vi "仁莫密封检测系统.vi"() -> ()   [LabVIEW 2020]
uses:
  <vilib>/event_ctls.llb/eventvkey.ctl
  <vilib>/NI/Modbus Library/API/Master/Modbus Master.lvclass
  <vilib>/Utility/file.llb/Read Delimited Spreadsheet (string).vi
  <vilib>/NI/Modbus Library/Transmission Data Unit/RTU/RTU Data Unit.lvclass
  <vilib>/NI/Modbus Library/Master Function Definition/Master Function Definition.lvclass
  <vilib>/NI/Modbus Library/Network Protocol/Network Master/Serial/Serial Master.lvclass
panel:
  in  "sn":string
  in  "扫码启动":bool
  out "MES状态":bool
  out "通讯状态":bool
  out "泄漏流量":string
  out "参数组别":string
  out "测试时间":string
  out "实时压力":string
  out "泄漏压力":string
  out "门限压力":string
  out "目标压力":string
  out "测试 NG":string
  out "测试 OK":string
  out "测试结果":string
  out "测试总量":string
  out "实时压力(图)":dbl(graph)
  out "消息框+":string
  in  "清除计数":bool
  in  "设备启动":bool
  out "运行状态":string
  in  "设备停止":bool
  in  "阻断通讯":bool=TRUE
  out "运行状态":string
  out "失败原因":string
  in  "Exit":bool
  # "仁 莫 密 封 检 测 系 统"
  # "sccm"
  # "S"
  # "Pa"
  # "Pa"
  # "Pa"
  # "Pa"
  # "pcs"
  # "pcs"
  # "pcs"
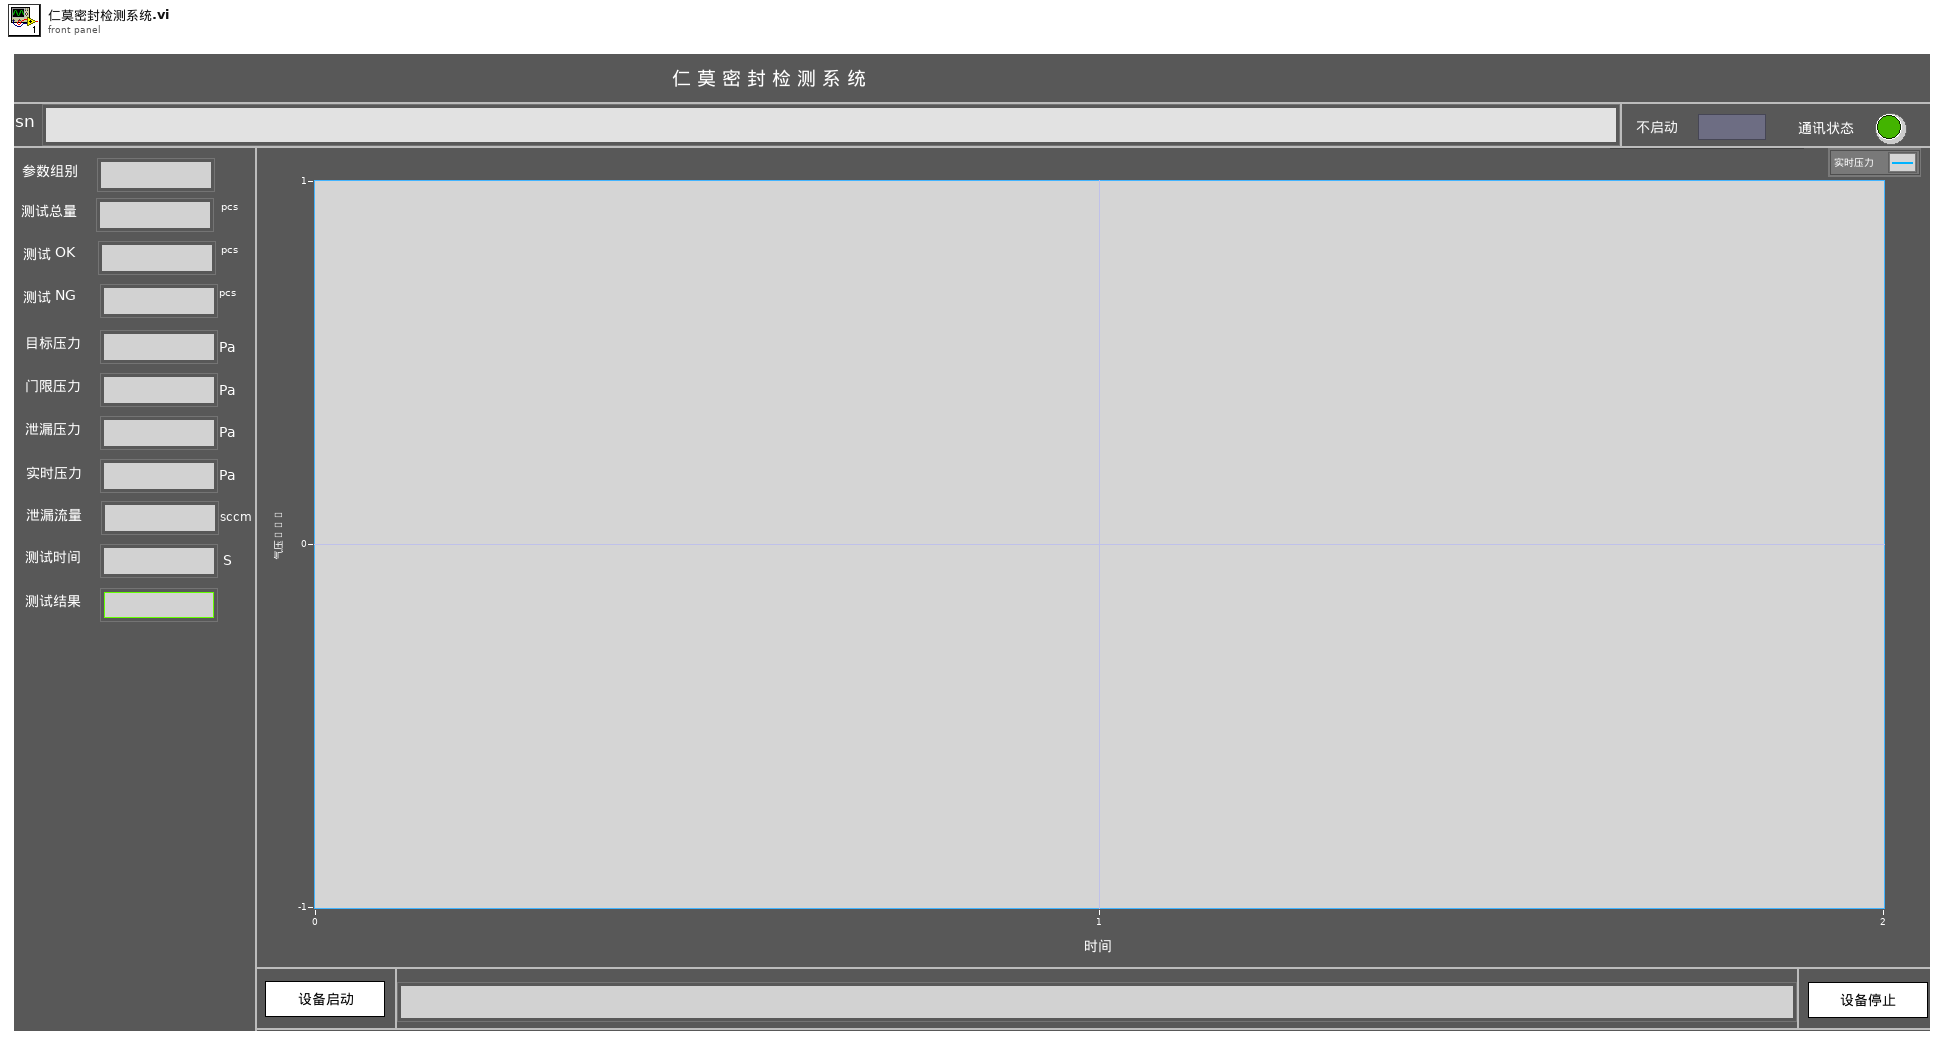
[diagram p1: front panel]
types:
  T1 = typedef "eventvkey.ctl" = enum16{"ASCII", "Enter", "Return", "Shift", "Ctrl", "Alt", "Cmd", "Opt", "Caps", "NumLock", "Clear", "Break", "Up", "Down", "Left", "Right", "Insert", "Delete", "Home", "End", "PageUp", "PageDown", "Escape", "Help", "Pause", "ScrollLock", "F1", "F2", "F3", "F4", "F5", "F6", "F7", "F8", "F9", "F10", "F11", "F12", "F13", "F14", "F15", "F16", "F17", "F18", "F19", "F20", "F21", "F22", "F23", "F24", "Play", "VolumeUp", "VolumeDown", "Mute", "Two Byte Char"}
  T2 = cluster{"地址":u16, "数量":u16, "寄存器值":u16[], "产品总数":string}[]
  T3 = enum32{"Invalid", "Standard", "Closed", "Hidden", "Minimized", "Maximized"}
  T4 = enum32{"invalid app kind", "Development System", "Run Time System", "Student Edition", "Embedded LabVIEW", "Evaluation", "Custom"}
  T5 = cluster{"地址":u16, "数量":u16, "寄存器值":u16[], "名称":string}[]
  T6 = cluster{"读取信息簇":cluster{"地址":u16, "数量":u16, "寄存器值":u16[], "名称":string}, "值解析":string}[]
  T7 = cluster{"温度instance":refnum<class "Modbus Master.lvclass">, "Core":cluster{"Current VI Reference":refnum<vi>, "Close Panel on Exit?":bool}, "serial master instance":refnum<class "Modbus Master.lvclass">, "进站OK":bool, "连接成功":bool, "正在运行":bool, "用户登录":bool, "A读保持寄存器信息组":cluster{"地址":u16, "数量":u16, "寄存器值":u16[], "名称":string}[], "A写入线圈信息组":cluster{"地址":u16, "布尔":bool, "名称":string}[], "A读多组线圈信息组":cluster{"地址":u16, "数量":u16, "名称":string, "线圈组":bool[]}[]}
  T8 = cluster{"连接成功":bool, "MB_实体":refnum<class "Modbus Master.lvclass">}
  T9 = cluster{"地址":u16, "数量":u16, "名称":string, "线圈组":bool[]}[]
  T10 = cluster{"Current VI Reference":refnum<vi>, "Close Panel on Exit?":bool}
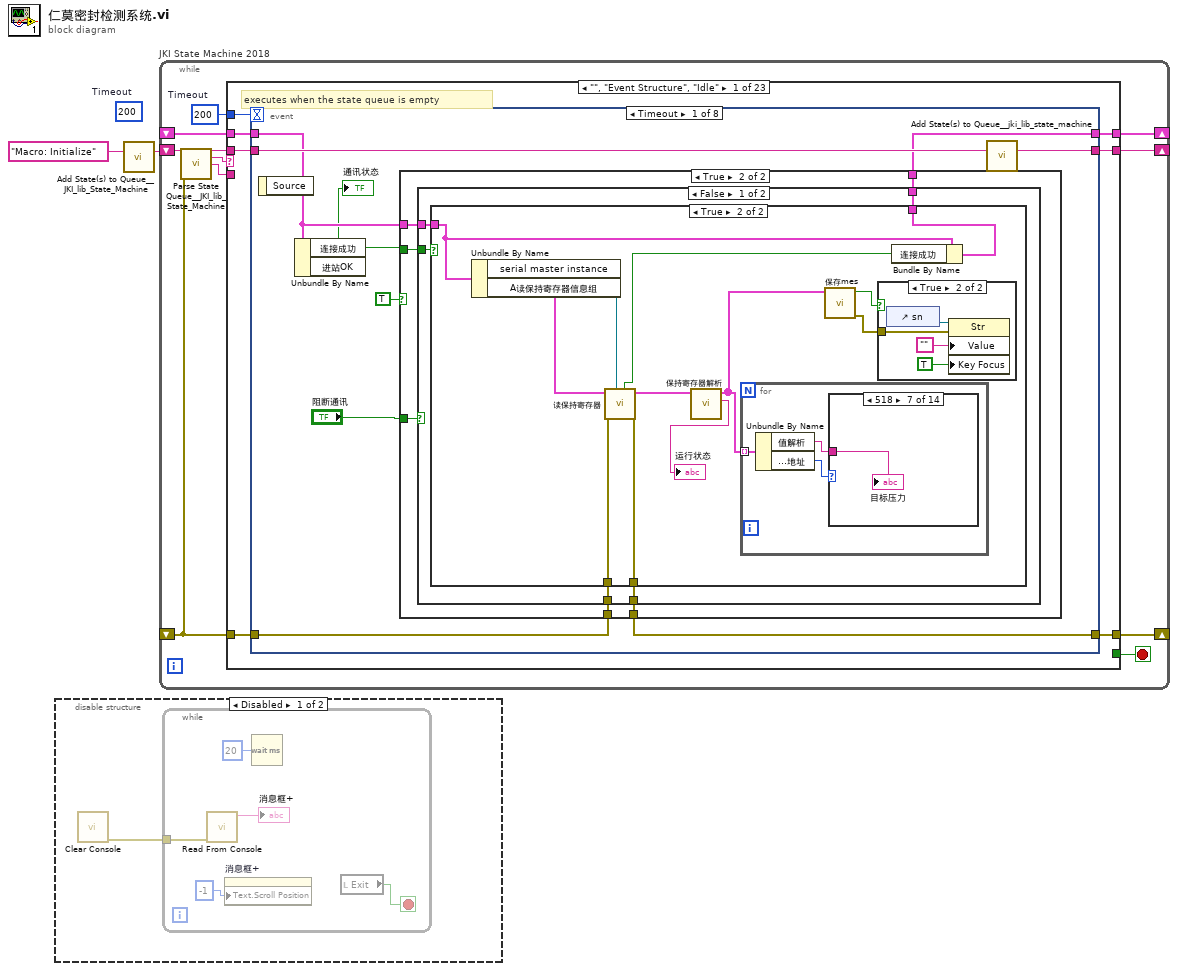
[diagram p0: block diagram]
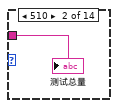
[diagram p7: hidden frame]
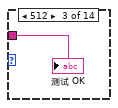
[diagram p8: hidden frame]
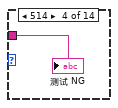
[diagram p9: hidden frame]
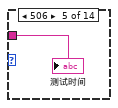
[diagram p10: hidden frame]
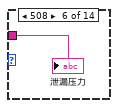
[diagram p11: hidden frame]
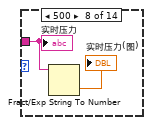
[diagram p12: hidden frame]
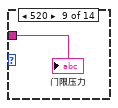
[diagram p13: hidden frame]
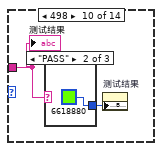
[diagram p14: hidden frame]
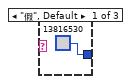
[diagram p15: hidden frame]
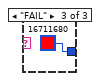
[diagram p16: hidden frame]
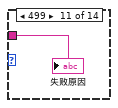
[diagram p17: hidden frame]
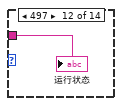
[diagram p18: hidden frame]
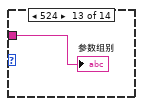
[diagram p19: hidden frame]
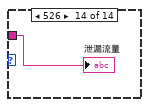
[diagram p20: hidden frame]
diagram:
  (unwired) 200  # Timeout
  n1 = disable-structure shown="Disabled" {
    frame Disabled {
      n2 = call "Clear Console.vi"() -> ("error out"=w3:errorcluster)  [unwired: 11 in]
      n3 = while {
        tunnel: w3 -> [w7]
        stop <- w4 stop-if-true
        n4 = call "Read From Console.vi"("error in (no error)"=w7) -> ("Output"=→"消息框+":string)  [unwired: 9 in, 1 out]
        n5 = property on="消息框+" class="Str"("Text.Scroll Position"=i8 -1 ("milliseconds to wait")) -> ()  [unwired: 2 in, 2 out]
        n6 = Wait (ms)(milliseconds to wait=u32 20 ("等待时间（毫秒）")) -> ()  [unwired: 1 out]
        n7 = local read "Exit"() -> (w4:bool)
      }
    }
    frame Enabled {
    }
  }
  n8 = call <vilib>:"Add State(s) to Queue__JKI_lib_State_Machine.vi"("State(s) in (\"\")"="Macro: Initialize") -> ("States Out"=w2:string)  [unwired: 14 in]
  n9 = while "JKI State Machine 2018" {
    shift-right: [w12] -> _
    shift-left: _ -> [w11]
    shift-right: [w15] -> _
    shift-left: _ -> [w9]
    shift-right: [w14] -> _
    shift-left: w2 -> [w16]
    stop <- w13 stop-if-true
    w10 = 200  # Timeout
    n10 = call <vilib>:"Parse State Queue__JKI_lib_State_Machine.vi"("State Queue"=w16, "Error In (no error)"=w9) -> ("Remaining States"=w18:string, "Current State"=w19:string, "Arguments"=w17:string)  [unwired: 11 in]
    n11 = case shown="\"\", \"Event Structure\", \"Idle\"" w19 {
      selector: w19 -> [_ _ w199 _ _ _ _ _ _ _ _ _ _ _ _ _ _ _ _ _ _ _ _]
      tunnel: w18 -> [w26 w198 w203 w222 w229 w234 w238 w263 w272 w276 w293 w299 w310 w379 w384 w394 w398 w410 w422 w469 w501 w513 w518]
      tunnel: w17 -> [_ _ _ _ _ _ _ _ _ _ _ w294 w304 _ _ _ _ _ _ _ _ _ _]
      tunnel: w11 -> [w24 w195 w201 w215 w226 w232 w235 _ w268 w273 w291 w297 w306 w376 w381 w391 w395 w404 w416 w463 w494 w510 w515]
      tunnel: [w23 w196 w205 w219 errorcluster {"status"=FALSE, "code"=0, "source"=""} ("error out") w231 w236 w260 w269 w274 w290 w295 w307 w377 w382 w392 w396 w399 w419 w466 w498 w511 w516] -> w15
      tunnel: w9 -> [w22 w196 w204 w219 w224 w231 w236 w260 w266 w274 w290 w296 w308 w377 w382 w392 w396 w407 w420 w467 w499 w511 w516]
      tunnel: [w25 w197 w202 w221 w228 w233 w237 w262 w271 w275 w292 w298 w309 w378 w383 w393 w397 w409 w421 w468 w500 w512 w517] -> w14
      tunnel: [_ _ _ _ _ w230 _ _ _ _ _ _ _ _ _ _ _ _ _ _ _ _ _] -> w13
      tunnel: [w21 w195 w201 w220 w226 w232 w235 w261 w268 w273 w291 w297 w306 w376 w381 w391 w395 w402 w414 w461 w495 w510 w514] -> w12
      tunnel: w10 -> [w20 _ _ _ _ _ _ _ _ _ _ _ _ _ _ _ _ _ _ _ _ _ _]
      frame "", "Event Structure", "Idle" {
        # "executes when the state queue is empty"
        n12 = event shown="[0] Timeout" {
          selector: _ -> [_ _ _ _ _ _ _ _]
          dyn-events: _ -> [_ _ _ _ _ _ _ _]
          timeout: w20 -> [_ _ _ _ _ _ _ _]
          tunnel: w26 -> [w35 w94 w99 w105 w159 w178 w188 w194]
          tunnel: [w34 w93 w98 w104 w158 w177 w187 w193] -> w25
          tunnel: w24 -> [w33 w91 w96 w101 w156 w173 w185 w191]
          tunnel: [w31 w92 w97 w103 w157 w170 w186 w192] -> w23
          tunnel: w22 -> [w32 w92 w97 w103 w157 w171 w186 w192]
          tunnel: [w30 w91 w96 w100 w156 w172 w185 w191] -> w21
          event Timeout {
            n13 = event-data() -> ()  [unwired: 1 in, 1 out]
            n14 = Unbundle By Name(w33) -> ("连接成功"=w27:bool)  [unwired: 1 out]
            "通讯状态" <- w27
            n15 = case shown="True" TRUE {
              tunnel: w33 -> [w37 w43]
              tunnel: w32 -> [w36 w42]
              tunnel: [w36 w41] -> w31
              tunnel: [w37 w40] -> w30
              tunnel: "阻断通讯" -> [_ w39]
              tunnel: w27 -> [_ w38]
              frame False {
              }
              frame True {
                n16 = case shown="False" w39 {
                  tunnel: w38 -> [w48 _]
                  tunnel: w43 -> [w47 w88]
                  tunnel: w42 -> [w46 w89]
                  tunnel: [w45 w89] -> w41
                  tunnel: [w44 w88] -> w40
                  frame False {
                    n17 = case shown="True" w48 {
                      tunnel: w47 -> [w49 w60]
                      tunnel: w46 -> [w50 w62]
                      tunnel: [w50 w61] -> w45
                      tunnel: [w49 w55] -> w44
                      frame False {
                      }
                      frame True {
                        n18 = Unbundle By Name(w60) -> ("serial master instance"=w59:refnum<class "Modbus Master.lvclass">, "A读保持寄存器信息组"=w58:T5)
                        n19 = call "读保持寄存器.vi"("MB_实体"=w59, "error in"=w62, "读保持寄存器信息组__输入"=w58) -> ("输出簇"=w61:errorcluster, "读保持寄存器信息组_输出"=w56:T5, "连接成功"=w57:bool)  [unwired: 6 in]
                        n20 = call "保持寄存器解析.vi"("A读保持寄存器信息组"=w56) -> ("运行状态"=→"运行状态":string, "参数值"=w54:T6)  [unwired: 9 in]
                        n21 = for {
                          tunnel: w54 -> [w68] mode=indexing
                          n22 = Unbundle By Name(w68) -> ("值解析"=w67:string, "读取信息簇.地址"=w69:u16)
                          n23 = case shown="518" w69 {
                            tunnel: w67 -> [_ w70 w71 w72 w73 w74 w75 w77 w78 w80 w84 w85 w86 w87]
                            frame Default {
                            }
                            frame 510 {
                              "测试总量" <- w70
                            }
                            frame 512 {
                              "测试 OK" <- w71
                            }
                            frame 514 {
                              "测试 NG" <- w72
                            }
                            frame 506 {
                              "测试时间" <- w73
                            }
                            frame 508 {
                              "泄漏压力" <- w74
                            }
                            frame 518 {
                              "目标压力" <- w75
                            }
                            frame 500 {
                              n24 = Fract/Exp String To Number(string=w77) -> (number=→"实时压力(图)":dbl)  [unwired: 3 in, 1 out]
                              "实时压力" <- w77
                            }
                            frame 520 {
                              "门限压力" <- w78
                            }
                            frame 498 {
                              n25 = case shown="\"PASS\"" w80 {
                                tunnel: [u32 13816530 ("颜色盒") u32 6618880 u32 16711680] -> w79
                                frame "假", Default {
                                }
                                frame "PASS" {
                                }
                                frame "FAIL" {
                                }
                              }
                              n26 = property on="测试结果" class="Str"("Text.BGColor"=w79) -> ()  [unwired: 2 in, 2 out]
                              "测试结果" <- w80
                            }
                            frame 499 {
                              "失败原因" <- w84
                            }
                            frame 497 {
                              "运行状态" <- w85
                            }
                            frame 524 {
                              "参数组别" <- w86
                            }
                            frame 526 {
                              "泄漏流量" <- w87
                            }
                          }
                        }
                        n27 = call "保存mes.vi"("参数值"=w54) -> ("error out"=w52:errorcluster, "出站成功"=w51:bool)  [unwired: 9 in]
                        n28 = case shown="True" w51 {
                          tunnel: w52 -> [_ w65]
                          frame False {
                          }
                          frame True {
                            n29 = control-ref of="sn"() -> (w66:refnum<vi>)
                            n30 = property on="属性节点" class="Str"(reference=w66, error in=w65, "Value"="", "Key Focus"=TRUE ("键选中")) -> ()  [unwired: 2 out]
                          }
                        }
                        n31 = Bundle By Name(cluster=w60, "连接成功"=w57) -> (w55:T7)
                      }
                    }
                  }
                  frame True {
                  }
                }
              }
            }
            n32 = call <vilib>:"Add State(s) to Queue__jki_lib_state_machine.vi"("State(s) in (\"\")"=w35) -> ("States Out"=w34:string)  [unwired: 14 in]
          }
          event "设备启动": Value Change {
            n33 = event-data() -> ()  [unwired: 1 in, 1 out]
            n34 = call <vilib>:"Add State(s) to Queue__jki_lib_state_machine.vi"("State(s) in Front (\"\")"="//Communication: 读运行标志\nCommunication: 设备启动\n//Communication: 读运行标志", "State(s) in (\"\")"=w94) -> ("States Out"=w93:string)  [unwired: 13 in]
          }
          event "设备停止": Value Change {
            n35 = event-data() -> ()  [unwired: 1 in, 1 out]
            n36 = call <vilib>:"Add State(s) to Queue__jki_lib_state_machine.vi"("State(s) in Front (\"\")"="//Communication: 读运行标志\nCommunication: 设备停止\n//Communication: 读运行标志", "State(s) in (\"\")"=w99) -> ("States Out"=w98:string)  [unwired: 13 in]
          }
          event Menu Selection (User) {
            n37 = event-data() -> ("ItemTag"=w102:string)  [unwired: 1 in]
            n38 = case shown="\"历史数据路径配置\"" w102 {
              tunnel: w101 -> [w106 w107 w118 w129 w130 w132 w143 w151]
              tunnel: [w106 w107 w118 w129 w130 w131 w142 w151] -> w100
              frame "假", Default {
              }
              frame "历史数据查询" {
                n39 = stacked-sequence {
                  frame #0 {
                    n40 = call <vilib>:"Check if File or Folder Exists.vi"("path"=path "D:/MES" ("路径")) -> ("file or folder exists?"=w110:bool, "dup path"=w109:path)  [unwired: 8 in, 1 out]
                    n41 = case shown="False" w110 {
                      tunnel: w109 -> [w112 w113]
                      tunnel: [w111 w113] -> _
                      frame False {
                        n42 = Create Folder(path (use dialog)=w112) -> (created path=w111:path)  [unwired: 2 in, 2 out]
                      }
                      frame True {
                      }
                    }
                  }
                  frame #1 {
                    n43 = call <vilib>:"Space Constant.vi"() -> ("String"=w115:string)
                    n44 = Concatenate Strings("explorer" ("字符串"), w115, "D:\\MES" ("字符串")) -> (w117:string)
                    n45 = call <vilib>:"System Exec.vi"("command line"=w117) -> ()  [unwired: 7 in, 4 out]
                  }
                }
              }
              frame "MES日志查询" {
                n46 = stacked-sequence {
                  frame #0 {
                    n47 = call <vilib>:"Check if File or Folder Exists.vi"("path"=path "D:/Log" ("路径")) -> ("file or folder exists?"=w121:bool, "dup path"=w120:path)  [unwired: 8 in, 1 out]
                    n48 = case shown="False" w121 {
                      tunnel: w120 -> [w123 w124]
                      tunnel: [w122 w124] -> _
                      frame False {
                        n49 = Create Folder(path (use dialog)=w123) -> (created path=w122:path)  [unwired: 2 in, 2 out]
                      }
                      frame True {
                      }
                    }
                  }
                  frame #1 {
                    n50 = call <vilib>:"Space Constant.vi"() -> ("String"=w126:string)
                    n51 = Concatenate Strings("explorer" ("字符串"), w126, "D:\\Log" ("字符串")) -> (w128:string)
                    n52 = call <vilib>:"System Exec.vi"("command line"=w128) -> ()  [unwired: 7 in, 4 out]
                  }
                }
              }
              frame "IP配置" {
                n53 = call "IP配置.vi"() -> ()  [unwired: 11 in, 1 out]
              }
              frame "历史数据路径配置" {
                n54 = call "Path配置.vi"() -> ()  [unwired: 11 in, 1 out]
              }
              frame "通讯参数设置" {
                n55 = stacked-sequence {
                  tunnel: w132 -> [_ w137 _]
                  tunnel: [_ w134 _] -> w131
                  frame #0 {
                    n56 = local write "阻断通讯"(TRUE ("阻断通讯")) -> ()
                  }
                  frame #1 {
                    n57 = call "通讯参数设置.vi"() -> ("A设备簇"=w138:T8)  [unwired: 5 in]
                    n58 = Unbundle By Name(w138) -> ("MB_实体"=w136:refnum<class "Modbus Master.lvclass">, "连接成功"=w135:bool)
                    n59 = Bundle By Name(cluster=w137, "serial master instance"=w136, "连接成功"=w135) -> (w134:T7)
                  }
                  frame #2 {
                    n60 = local write "阻断通讯"(FALSE ("阻断通讯")) -> ()
                  }
                }
              }
              frame "本地控制" {
                n61 = call "本地控制.vi"() -> ("远程2"=w141:bool)  [unwired: 11 in]
                "MES状态" <- w141
                n62 = Not(x=w141) -> (.not. x?=w140:bool)
                n63 = Bundle By Name(cluster=w143, "用户登录"=w140, "进站OK"=w140) -> (w142:T7)
                n64 = global write "Global.vi" "产品进站"(w140) -> ()
                n65 = case shown="True" w141 {
                  frame False {
                    n66 = Current VI's Menubar() -> (w145:refnum<k9>)
                    n67 = Delete Menu Items(9:w145) -> (3:w144:refnum<k9>)  [unwired: 3 in, 1 out]
                    n68 = Insert Menu Items(7:string[] ["历史数据查询", "通讯参数设置", "MES配置", "MES日志查询", "本地控制", "温湿度设置"] ("L10n_item tags 1"), 9:w144) -> ()  [unwired: 4 in, 3 out]
                  }
                  frame True {
                    n69 = Current VI's Menubar() -> (w149:refnum<k9>)
                    n70 = Delete Menu Items(9:w149) -> (0:w147:errorcluster, 3:w148:refnum<k9>)  [unwired: 3 in]
                    n71 = Insert Menu Items(6:w147, 7:string[] ["用户登录", "历史数据查询", "通讯参数设置", "MES配置", "MES日志查询", "本地控制", "温湿度设置"] ("L10n_item tags 1"), 9:w148) -> ()  [unwired: 3 in, 3 out]
                  }
                }
              }
              frame "机台号设置" {
                n72 = call "机台号设置.vi"() -> ()  [unwired: 11 in, 1 out]
              }
            }
            n73 = call <vilib>:"Add State(s) to Queue__jki_lib_state_machine.vi"("State(s) in (\"\")"=w105) -> ("States Out"=w104:string)  [unwired: 14 in]
          }
          event "sn": Key Down {
            # "20221205\n屏蔽扫码启动功能\n20221214\n既可以扫码启动也可以直接启动\n20230321\n扫码显示机台号\n20230323\n扫码，加机台号"
            n74 = event-data() -> ("VKey"=w155:T1)  [unwired: 1 in]
            n75 = Equal?(x=w155, y=eventvkey."Return" ("V键")) -> (x = y?=w153:bool)
            n76 = case shown="True" w153 {
              tunnel: [_ w166] -> w152
              frame False {
              }
              frame True {
                w162 = ""
                n77 = case shown="True" "扫码启动" {
                  tunnel: ["" "Communication: 设备启动"] -> w166
                  frame False {
                  }
                  frame True {
                  }
                }
                n78 = Search and Replace String(input string="sn", search string="\n", replace string=w162) -> (result string=w165:string)  [unwired: 5 in, 3 out]
                n79 = Search and Replace String(input string=w165, search string="\r", replace string=w162) -> (result string=w160:string)  [unwired: 5 in, 3 out]
                n80 = global write "Global.vi" "sn"(w160) -> ()
              }
            }
            n81 = call <vilib>:"Add State(s) to Queue__jki_lib_state_machine.vi"("State(s) in (\"\")"=w159, "State(s) at Back (\"\")"=w152) -> ("States Out"=w158:string)  [unwired: 13 in]
          }
          event "清除计数": Value Change {
            n82 = event-data() -> ()  [unwired: 1 in, 1 out]
            n83 = local write "清除计数"(FALSE) -> ()
            n84 = Unbundle By Name(w173) -> ("serial master instance"=w174:refnum<class "Modbus Master.lvclass">)
            n85 = disable-structure shown="禁用" {
              disable-tunnel: [w183 _] -> w175
              disable-tunnel: w174 -> [w182 _]
              disable-tunnel: w171 -> [w180 _]
              disable-tunnel: [w179 _] -> w170
              frame Disabled {
                n86 = call "写保持寄存器.vi"("MB_实体"=w182, "error in"=w180, "读保持寄存器信息组__输入"=T2 [{"地址"=510, "数量"=2, "寄存器值"=[0, 0], "产品总数"="产品总数"}, {"地址"=512, "数量"=2, "寄存器值"=[0, 0], "产品总数"="合格数量"}, {"地址"=514, "数量"=2, "寄存器值"=[0, 0], "产品总数"="泄露数量"}]) -> ("输出簇"=w179:errorcluster, "连接成功"=w183:bool)  [unwired: 7 in]
              }
              frame Enabled {
              }
            }
            n87 = Bundle By Name(cluster=w173, "连接成功"=w175) -> (w172:T7)
            n88 = call <vilib>:"Add State(s) to Queue__jki_lib_state_machine.vi"("State(s) in (\"\")"=w178) -> ("States Out"=w177:string)  [unwired: 14 in]
          }
          event "Exit": Value Change {
            # "Exit Button Value Change (pressed) Event\n(this executes Macro: Exit to terminate the VI)"
            n89 = event-data() -> ()  [unwired: 1 in, 1 out]
            n90 = call <vilib>:"Add State(s) to Queue__jki_lib_state_machine.vi"("State(s) in Front (\"\")"="Macro: Exit", "State(s) in (\"\")"=w188) -> ("States Out"=w187:string)  [unwired: 13 in]
          }
          event Panel Close? {
            # "Discard the event because we'll close the front panel ourselves in Macro: Exit"
            # "Close Panel button (pressed) Event\n(this executes Macro: Exit to terminate the VI)"
            n91 = event-data() -> ()  [unwired: 1 in, 1 out]
            n92 = call <vilib>:"Add State(s) to Queue__jki_lib_state_machine.vi"("State(s) in Front (\"\")"="Macro: Exit", "State(s) in (\"\")"=w194) -> ("States Out"=w193:string)  [unwired: 13 in]
            n93 = event-data("Discard?"=TRUE) -> ()  [unwired: 1 in, 1 out]
          }
        }
      }
      frame "---------- Core ----------" {
        # "Do not put any code in this frame.\n(it is a separator no-op)"
        n94 = call <vilib>:"Add State(s) to Queue__jki_lib_state_machine.vi"("State(s) in (\"\")"=w198) -> ("States Out"=w197:string)  [unwired: 14 in]
      }
      frame Default {
        w208 = 42 items=["No error", "Argument error", "Memory is full", "Out of zone", "End of file", "File already open", "Generic file I/O error", "File not found", "File permission error", "Disk is full", "Duplicate path", "Too many files open", "System feature not enabled", "Resource file not found", "Cannot add resource", "Resource not found", "Image not found", "Image memory error", "Pen does not exist", "Config type invalid", "Config token not found", "Config parse error", "Config memory error", "Bad external code format", "Bad external code offset", "External code not present", "Null window", "Destroy window error", "Null menu", "Print aborted", "Bad print record", "Print driver error", "Windows error during printing", "Memory error during printing", "Print dialog error", "Generic print error", "Invalid device refnum", "Device not found", "Device parameter error", "Device unit error", "Cannot open device", "Device call aborted", "Generic error", "Cancelled by user", "Object ID too low", "Object ID too high", "Object not in heap", "Unknown heap", "Unknown object (invalid DefProc)", "Unknown object (DefProc not in table)", "Message out of range", "Invalid (null) method", "Unknown message", "Manager call not supported", "Bad address", "Network operation in progress", "Network operation timed out", "Connection is busy", "Network attribute not supported", "Network error", "Address in use", "System out of memory", "Connection aborted", "Connection refused", "Not connected", "Already connected", "Connection closed", "Initialization error (interapplication manager)", "Bad occurrence", "Wait on unbound occurrence handler", "Occurrence queue overflow", "Datalog type conflict", "Unused", "Unrecognized type (interapplication manager)", "Memory corrupt", "Failed to make temporary DLL", "Old CIN version", "Drag socket not found", "Failed to load drop-object", "Failed to register OLE object", "Failed to release OLE object", "Format specifier type mismatch", "Unknown format specifier", "Too few format specifiers", "Too many format specifiers", "Scan failed", "Newer CIN version", "Error converting to variant", "Runtime menu error", "Password tampered", "Variant attribute not found", "Incompatible variant data type", "Event data is not available", "Event Store is not present", "Occurrence is not found", "Event Queue is not created", "Event info is not available", "Refnum passed is NULL", "Error retrieving Class GUID", "Error retrieving CoClass GUID", "Error retrieving TypeLib GUID.", "Bad built application magic bytes.", "Specific driver is different from the specific driver associated with the Logical Name.", "There is no session opened to the class driver.", "Max Error", "MAX - Error with config objects", "MAX - Error loading configuration", "MAX - Group not supported"]
        # "Current State"
        # "Do not delete, rename, or modify this frame.\n(this is used to capture unhandled states and typos)"
        # "Handle mistyped state name (developer tool)"
        n95 = Format Into String(format string="Software Exception: Unhandled State \"%s\"." ("message"), error in=w204, w199) -> (resulting string=w207:string, error out=w206:errorcluster)  [unwired: 1 in]
        n96 = call <vilib>:"Error Cluster From Error Code.vi"("show call chain? (False)"=TRUE, "error in (no error)"=w206, "error message (\"\")"=w207, "error code (0)"=w208) -> ("error out"=w205:errorcluster)  [unwired: 5 in]
        n97 = call <vilib>:"Add State(s) to Queue__jki_lib_state_machine.vi"("State(s) in (\"\")"=w203) -> ("States Out"=w202:string)  [unwired: 14 in]
      }
      frame "Initialize Core Data" {
        # "Do not delete, rename, or modify this frame.\n(this is used to determine panel behavior on exit)"
        # "originally closed?"
        # "exe?"
        # "If panel starts closed or is an EXE, then close it when we exit"
        n98 = property class="VI"() -> ("FP.State"=w212:T3)  [unwired: 2 in, 2 out]
        n99 = property class="App"() -> ("App.Kind"=w218:T4)  [unwired: 2 in, 2 out]
        n100 = control-ref of="Current VI Reference"() -> (w213:refnum<vi>)
        n101 = Equal?(x=w212, y=T3."Closed" ("Front Panel Window:State")) -> (x = y?=w210:bool)
        n102 = Equal?(x=w218, y=T4."Run Time System" ("Application:Kind")) -> (x = y?=w216:bool)
        n103 = Or(x=w210, y=w216) -> (x .or. y?=w214:bool)
        n104 = Bundle By Name(cluster=w215, "Core.Current VI Reference"=w213, "Core.Close Panel on Exit?"=w214) -> (w220:T7)
        n105 = call <vilib>:"Add State(s) to Queue__jki_lib_state_machine.vi"("State(s) in (\"\")"=w222) -> ("States Out"=w221:string)  [unwired: 14 in]
      }
      frame "Error Handler" {
        # "Handle any errors here.\nYou can also output any states to clean-up after errors occur"
        # "Clear error"
        n106 = Unbundle By Name(w224) -> ("source"=w223:string)
        n107 = One Button Dialog(message=w223) -> ()  [unwired: 1 in, 1 out]
        n108 = call <vilib>:"Add State(s) to Queue__jki_lib_state_machine.vi"("State(s) in Front (\"\")"="/* Post Error States", "State(s) in (\"\")"=w229) -> ("States Out"=w228:string)  [unwired: 13 in]
      }
      frame "Exit" {
        w230 = TRUE
        # "Do not put any code in this frame.\n(No errors that occur here will be handled.)"
        n109 = local write "Exit"(w230) -> ()
        n110 = call <vilib>:"Add State(s) to Queue__jki_lib_state_machine.vi"("State(s) in (\"\")"=w234) -> ("States Out"=w233:string)  [unwired: 14 in]
      }
      frame "---------- Data ----------" {
        # "Do not put any code in this frame.\n(It is a separator no-op. You can make a copy of this frame to create a new Data frame)"
        n111 = call <vilib>:"Add State(s) to Queue__jki_lib_state_machine.vi"("State(s) in (\"\")"=w238) -> ("States Out"=w237:string)  [unwired: 14 in]
      }
      frame "Data: Initialize" {
        (unwired) FALSE ("产品进站")
        (unwired) FALSE  # 进站OK
        w243 = refnum<class "Modbus Master.lvclass"> refnum  # 温度instance
        w245 = TRUE  # 进站OK
        w252 = TRUE  # 用户登录
        w253 = FALSE  # 正在运行
        w254 = T5 [{"地址"=510, "数量"=2, "寄存器值"=[0, 0], "名称"="产品总数"}, {"地址"=512, "数量"=2, "寄存器值"=[0, 0], "名称"="合格数量"}, {"地址"=514, "数量"=2, "寄存器值"=[0, 0], "名称"="泄露数量"}, {"地址"=506, "数量"=2, "寄存器值"=[0, 0], "名称"="1测试时间"}, {"地址"=508, "数量"=2, "寄存器值"=[0, 0], "名称"="1测试泄漏"}, {"地址"=518, "数量"=2, "寄存器值"=[0, 0], "名称"="1#目标压力"}, {"地址"=498, "数量"=1, "寄存器值"=[0, 0], "名称"="1#测试结果"}, {"地址"=500, "数量"=2, "寄存器值"=[0, 0], "名称"="实时压力"}, {"地址"=520, "数量"=2, "寄存器值"=[], "名称"="门限压力"}, {"地址"=499, "数量"=1, "寄存器值"=[], "名称"="失败原因"}, {"地址"=497, "数量"=1, "寄存器值"=[], "名称"="运行状态"}, {"地址"=524, "数量"=2, "寄存器值"=[], "名称"="参数组别"}, {"地址"=526, "数量"=4, "寄存器值"=[], "名称"="泄漏流量"}]  # A读保持寄存器信息组
        w255 = T9 [{"地址"=507, "数量"=1, "名称"="1测试结束标志", "线圈组"=[FALSE, TRUE]}]  # A读多组线圈信息组
        w256 = cluster{"地址":u16, "布尔":bool, "名称":string}[] [{"地址"=50, "布尔"=FALSE, "名称"="启动"}, {"地址"=51, "布尔"=FALSE, "名称"="停止"}]  # A写入线圈信息组
        w257 = FALSE  # 连接成功
        w258 = refnum<class "Modbus Master.lvclass"> refnum  # serial master instance
        w259 = T10 {"Current VI Reference"=refnum, "Close Panel on Exit?"=FALSE}  # Core
        # "Initialize the shift-register data, here.\n(data names are defined by what you wire into the bundle function)"
        n112 = call <vilib>:"Application Directory.vi"() -> ("Application Directory"=w250:path)
        n113 = Build Path(base path=w250, name or relative path=path "data/mes.cfg") -> (appended path=w251:path)
        n114 = global write "Global.vi" "保存条件1"(FALSE ("保存条件1")) -> ()
        n115 = call "FGV_Boolean.vi"("点亮"=FALSE, "状态"=enum16{"Init", "Read", "Write"}."Init") -> ()  [unwired: 8 in, 2 out]
        n116 = call-poly <vilib>:"Read Delimited Spreadsheet.vi"("file path (dialog if empty)"=w251, "delimiter (\\t)"="::" ("delimiter (\\t)")) -> ("all rows"=w246:string[][])  [unwired: 8 in, 5 out]
        n117 = call "mes初始化.vi"("mes"=w246) -> ()  [unwired: 11 in]
        n118 = disable-structure shown="禁用" {
          frame Disabled {
            n119 = global write "Global.vi" "MES状态"(TRUE ("MES状态")) -> ()
          }
          frame Enabled {
          }
        }
        n120 = global write "Global.vi" "正在运行"(FALSE ("MES状态")) -> ()
        n121 = global write "Global.vi" "产品进站"(TRUE ("产品进站")) -> ()
        n122 = global write "Global.vi" "运行状态时间点"(dbl[] [0.0, 0.0, 0.0, 0.0, 0.0, 0.0, 0.0, 0.0, 0.0] ("运行状态时间点")) -> ()
        n123 = Bundle("温度instance"=w243, "Core"=w259, "serial master instance"=w258, "进站OK"=w245, "连接成功"=w257, "正在运行"=w253, "用户登录"=w252, "A读保持寄存器信息组"=w254, "A写入线圈信息组"=w256, "A读多组线圈信息组"=w255) -> (w261:T7)  [unwired: 1 in]
        n124 = call <vilib>:"Add State(s) to Queue__jki_lib_state_machine.vi"("State(s) in (\"\")"=w263) -> ("States Out"=w262:string)  [unwired: 14 in]
      }
      frame "Data: Cleanup" {
        # "Cleanup any data and references, here.\n(this is called automatically, by the Macro: Exit)"
        n125 = Unbundle By Name(w268) -> ("Core.Current VI Reference"=w270:refnum<vi>, "serial master instance"=w267:refnum<class "Modbus Master.lvclass">)
        n126 = call-dynamic "Shutdown.vi"("error in"=w266, "Modbus master in"=w267) -> ("error out"=w265:errorcluster)  [unwired: 9 in]
        n127 = Close Reference(reference=w270, error in (no error)=w265) -> (error out=w269:errorcluster)
        n128 = call <vilib>:"Add State(s) to Queue__jki_lib_state_machine.vi"("State(s) in (\"\")"=w272) -> ("States Out"=w271:string)  [unwired: 14 in]
      }
      frame "---------- UI ----------" {
        # "Do not put any code in this frame.\n(It is a separator no-op. You can make a copy of this frame to create a new UI frame)"
        n129 = call <vilib>:"Add State(s) to Queue__jki_lib_state_machine.vi"("State(s) in (\"\")"=w276) -> ("States Out"=w275:string)  [unwired: 14 in]
      }
      frame "UI: Initialize" {
        (unwired) string[] ["通讯参数设置", "IP配置", "历史数据路径配置"] ("L10n_item tags 1")
        # "Initialize the User Interface, here.\n(this is called automatically, by the Macro: Init)"
        n130 = call "读取配置文件.vi"("配置"="机台号") -> ("error out"=w279:errorcluster, "路径"=w277:string)  [unwired: 9 in]
        n131 = global write "Global.vi" "机台号"(w277) -> ()
        n132 = call "读取配置文件.vi"("error in"=w279, "配置"="程序名") -> ("error out"=w286:errorcluster, "路径"=w285:string)  [unwired: 8 in]
        n133 = local write "sn"("") -> ()
        n134 = property class="VI"(error in=w286, "Front Panel.Title"=w285) -> (error out=w283:errorcluster)  [unwired: 1 in, 1 out]
        n135 = Current VI's Menubar() -> (w289:refnum<k9>)
        n136 = Delete Menu Items(6:w283, 9:w289) -> (0:w288:errorcluster, 3:w287:refnum<k9>)  [unwired: 2 in]
        n137 = property on="测试结果" class="Str"("Text.BGColor"=u32 13816530 ("颜色盒")) -> ()  [unwired: 2 in, 2 out]
        n138 = Insert Menu Items(6:w288, 7:string[] ["通讯参数设置", "历史数据路径配置", "机台号设置"] ("L10n_item tags 1"), 9:w287) -> ()  [unwired: 3 in, 3 out]
        n139 = call <vilib>:"Add State(s) to Queue__jki_lib_state_machine.vi"("State(s) in (\"\")"=w293) -> ("States Out"=w292:string)  [unwired: 14 in]
      }
      frame "UI: Cursor Set" {
        # "Argument"
        # "Set and Unset Cursor Busy.\n(Usage: \"UI: Cursor Set >> Busy|Idle\")"
        n140 = case shown="\"Idle\", Default" w294 {
          tunnel: w296 -> [w301 w303]
          tunnel: [w300 w302] -> w295
          frame "Idle", Default {
            n141 = call <vilib>:"Unset Busy.vi"("error in (no error)"=w301) -> ("error out"=w300:errorcluster)  [unwired: 10 in]
          }
          frame "Busy" {
            n142 = call <vilib>:"Set Busy.vi"("error in (no error)"=w303) -> ("error out"=w302:errorcluster)  [unwired: 9 in, 1 out]
          }
        }
        n143 = call <vilib>:"Add State(s) to Queue__jki_lib_state_machine.vi"("State(s) in (\"\")"=w299) -> ("States Out"=w298:string)  [unwired: 14 in]
      }
      frame "UI: Front Panel State" {
        # "Argument"
        # "Set Front Panel Open or Closed\n(Usage: \"UI: Front Panel State >> Open|Close\")"
        n144 = Unbundle By Name(w306) -> ("Core.Current VI Reference"=w305:refnum<vi>)
        n145 = case shown="\"Maximize\", \"Maximized\"" w304 {
          tunnel: w308 -> [w316 w331 w342 w355 w368]
          tunnel: [w318 w332 w344 w357 w370] -> w307
          tunnel: w305 -> [w317 w329 w343 w356 w369]
          frame "Open", "Standard", Default {
            w311 = T3."Standard" ("State")
            n146 = property class="VI"(reference=w317, error in=w316) -> (reference out=w314:refnum<vi>, error out=w315:errorcluster, "FP.State"=w313:T3)
            n147 = Not Equal?(x=w313, y=w311) -> (x != y?=w312:bool)
            n148 = case shown="True" w312 {
              tunnel: [w322 w324] -> w318
              tunnel: w315 -> [w321 w324]
              tunnel: w314 -> [w320 _]
              tunnel: w311 -> [w319 _]
              frame True {
                n149 = invoke class="VI" method="FP.Open"(reference=w320, error in=w321, "Activate"=TRUE, "State"=w319) -> (error out=w322:errorcluster)  [unwired: 1 in, 4 out]
              }
              frame False {
              }
            }
          }
          frame "Close", "Closed" {
            n150 = property class="VI"(reference=w329, error in=w331) -> (reference out=w328:refnum<vi>, error out=w330:errorcluster, "FP.State"=w326:T3)
            n151 = Not Equal?(x=w326, y=T3."Closed" ("Front Panel Window:State")) -> (x != y?=w325:bool)
            n152 = case shown="True" w325 {
              tunnel: [w333 w336] -> w332
              tunnel: w330 -> [w333 w335]
              tunnel: w328 -> [_ w334]
              frame False {
              }
              frame True {
                n153 = invoke class="VI" method="FP.Close"(reference=w334, error in=w335) -> (error out=w336:errorcluster)  [unwired: 1 in, 2 out]
              }
            }
          }
          frame "Hidden", "Hide" {
            w337 = T3."Hidden" ("State")
            n154 = property class="VI"(reference=w343, error in=w342) -> (reference out=w340:refnum<vi>, error out=w341:errorcluster, "FP.State"=w339:T3)
            n155 = Not Equal?(x=w339, y=w337) -> (x != y?=w338:bool)
            n156 = case shown="True" w338 {
              tunnel: [w348 w349] -> w344
              tunnel: w341 -> [w347 w349]
              tunnel: w340 -> [w346 _]
              tunnel: w337 -> [w345 _]
              frame True {
                n157 = invoke class="VI" method="FP.Open"(reference=w346, error in=w347, "State"=w345) -> (error out=w348:errorcluster)  [unwired: 2 in, 4 out]
              }
              frame False {
              }
            }
          }
          frame "Minimize", "Minimized" {
            w350 = T3."Minimized" ("State")
            n158 = property class="VI"(reference=w356, error in=w355) -> (reference out=w353:refnum<vi>, error out=w354:errorcluster, "FP.State"=w352:T3)
            n159 = Not Equal?(x=w352, y=w350) -> (x != y?=w351:bool)
            n160 = case shown="True" w351 {
              tunnel: [w361 w362] -> w357
              tunnel: w354 -> [w360 w362]
              tunnel: w353 -> [w359 _]
              tunnel: w350 -> [w358 _]
              frame True {
                n161 = invoke class="VI" method="FP.Open"(reference=w359, error in=w360, "State"=w358) -> (error out=w361:errorcluster)  [unwired: 2 in, 4 out]
              }
              frame False {
              }
            }
          }
          frame "Maximize", "Maximized" {
            w363 = T3."Maximized" ("State")
            n162 = property class="VI"(reference=w369, error in=w368) -> (reference out=w366:refnum<vi>, error out=w367:errorcluster, "FP.State"=w365:T3)
            n163 = Not Equal?(x=w365, y=w363) -> (x != y?=w364:bool)
            n164 = case shown="True" w364 {
              tunnel: [w374 w375] -> w370
              tunnel: w367 -> [w373 w375]
              tunnel: w366 -> [w372 _]
              tunnel: w363 -> [w371 _]
              frame True {
                n165 = invoke class="VI" method="FP.Open"(reference=w372, error in=w373, "State"=w371) -> (error out=w374:errorcluster)  [unwired: 2 in, 4 out]
              }
              frame False {
              }
            }
          }
        }
        n166 = call <vilib>:"Add State(s) to Queue__jki_lib_state_machine.vi"("State(s) in (\"\")"=w310) -> ("States Out"=w309:string)  [unwired: 14 in]
      }
      frame "---------- Macro ----------" {
        # "Do not put any code in this frame.\n(It is a separator no-op. You can make a copy of this frame to create a new Macro frame)"
        n167 = call <vilib>:"Add State(s) to Queue__jki_lib_state_machine.vi"("State(s) in (\"\")"=w379) -> ("States Out"=w378:string)  [unwired: 14 in]
      }
      frame "Macro: Initialize" {
        w380 = "Data: Initialize\nInitialize Core Data\nUI: Initialize\nUI: Front Panel State >> Maximize\nCommunication: Open Serial\nCommunication: 读运行标志"  # Data: Initialize Initialize Core Data UI: Initialize UI: Front Panel State >> Maximize Communication: Open Serial Communication: 读运行标志
        # "Initialization Macro\n(This is called once, when the VI starts)"
        n168 = call <vilib>:"Add State(s) to Queue__jki_lib_state_machine.vi"("State(s) in Front (\"\")"=w380, "State(s) in (\"\")"=w384) -> ("States Out"=w383:string)  [unwired: 13 in]
      }
      frame "Macro: Exit" {
        # "Exit Macro\n(This is called once, when the VI exits)"
        n169 = Unbundle By Name(w391) -> ("Core.Close Panel on Exit?"=w390:bool)
        n170 = Select(t="UI: Front Panel State >> Close", s=w390, f="") -> (s? t:f=w387:string)
        n171 = call <vilib>:"Add State(s) to Queue__jki_lib_state_machine.vi"("State(s) in (\"\")"=w387, "State(s) at Back (\"\")"="Data: Cleanup\nExit") -> ("States Out"=w385:string)  [unwired: 13 in]
        n172 = call <vilib>:"Add State(s) to Queue__jki_lib_state_machine.vi"("State(s) in Front (\"\")"=w385, "State(s) in (\"\")"=w394) -> ("States Out"=w393:string)  [unwired: 13 in]
      }
      frame "---------- Communication ----------" {
        # "Template Separator\n(You can make a copy of, or modify, this frame)"
        n173 = call <vilib>:"Add State(s) to Queue__jki_lib_state_machine.vi"("State(s) in (\"\")"=w398) -> ("States Out"=w397:string)  [unwired: 14 in]
      }
      frame "Communication: Open Serial" {
        # "Your code here.\n(You can make a copy of, or modify, this frame)"
        n174 = call "读取配置文件.vi"("error in"=w407, "配置"="串口号") -> ("error out"=w406:errorcluster, "路径"=w405:string)  [unwired: 8 in]
        n175 = call "开机连接.vi"("error in"=w406, "波特率"=u32 19200, "串口号"=w405) -> ("error out"=w399:errorcluster, "连接成功"=w401:bool, "serial master instance"=w403:refnum<class "Modbus Master.lvclass">)  [unwired: 6 in]
        n176 = Bundle By Name(cluster=w404, "serial master instance"=w403, "连接成功"=w401) -> (w402:T7)
        n177 = call <vilib>:"Add State(s) to Queue__jki_lib_state_machine.vi"("State(s) in (\"\")"=w410) -> ("States Out"=w409:string)  [unwired: 14 in]
      }
      frame "Communication: 设备启动" {
        # "Your code here.\n(You can make a copy of, or modify, this frame)"
        n178 = Unbundle By Name(w416) -> ("serial master instance"=w417:refnum<class "Modbus Master.lvclass">, "连接成功"=w418:bool, "进站OK"=w411:bool)
        n179 = case shown="True" w411 {
          tunnel: w420 -> [w424 w434]
          tunnel: [w424 w433] -> w419
          tunnel: w418 -> [w425 w432]
          tunnel: w417 -> [_ w431]
          tunnel: [w425 w430] -> w415
          tunnel: FALSE ("正在运行") -> [w426 w429]
          tunnel: [w426 w428] -> w412
          tunnel: w411 -> [w423 _]
          frame False {
            n180 = case shown="False" w423 {
              frame False {
                n181 = One Button Dialog(message="产品未进站。" ("消息")) -> ()  [unwired: 1 in, 1 out]
              }
              frame True {
              }
            }
          }
          frame True {
            n182 = case shown="False" w429 {
              selector: w429 -> [_ w456]
              tunnel: w434 -> [w440 w457]
              tunnel: [w439 w457] -> w433
              tunnel: w432 -> [w438 w458]
              tunnel: w431 -> [w437 _]
              tunnel: [w436 w458] -> w430
              tunnel: [w435 w456] -> w428
              frame False {
                n183 = case shown="True" w438 {
                  tunnel: w440 -> [w441 w446]
                  tunnel: [w441 w445] -> w439
                  tunnel: w437 -> [_ w444]
                  tunnel: [_ w443] -> w436
                  tunnel: [_ TRUE] -> w435
                  frame False {
                  }
                  frame True {
                    n184 = stacked-sequence {
                      tunnel: w446 -> [_ w452 _ _]
                      tunnel: [_ w451 _ _] -> w445
                      tunnel: w444 -> [_ w450 _ _]
                      tunnel: [_ w449 _ _] -> w443
                      frame #0 {
                        n185 = local write "阻断通讯"(TRUE ("阻断通讯")) -> ()
                      }
                      frame #1 {
                        w448 = cluster{"地址":u16, "布尔":bool, "名称":string}[] [{"地址"=50, "布尔"=TRUE, "名称"="启动"}, {"地址"=51, "布尔"=FALSE, "名称"="停止"}]  # A写入线圈信息组
                        n186 = call "写入单个线圈.vi"("error in"=w452, "写入线圈信息组"=w448, "MB_实体"=w450) -> ("输出簇"=w451:errorcluster, "连接成功"=w449:bool)  [unwired: 7 in]
                      }
                      frame #2 {
                        n187 = local write "阻断通讯"(FALSE ("阻断通讯")) -> ()
                      }
                      frame #3 {
                        n188 = Format Date/Time String(time format string (%c)="%Y-%m-%d %H:%M:%S" ("EndTime")) -> (date/time string=w454:string)  [unwired: 2 in]
                        n189 = global write "Global.vi" "start_time"(w454) -> ()
                      }
                    }
                  }
                }
              }
              frame True {
              }
            }
          }
        }
        n190 = Bundle By Name(cluster=w416, "正在运行"=w412, "连接成功"=w415) -> (w414:T7)
        n191 = call <vilib>:"Add State(s) to Queue__jki_lib_state_machine.vi"("State(s) in (\"\")"=w422) -> ("States Out"=w421:string)  [unwired: 14 in]
      }
      frame "Communication: 设备停止" {
        # "Your code here.\n(You can make a copy of, or modify, this frame)"
        n192 = Unbundle By Name(w463) -> ("serial master instance"=w464:refnum<class "Modbus Master.lvclass">, "连接成功"=w465:bool)
        n193 = case shown="True" TRUE ("正在运行") {
          selector: TRUE ("正在运行") -> [w470 _]
          tunnel: w467 -> [w471 w478]
          tunnel: [w471 w477] -> w466
          tunnel: w465 -> [w472 w476]
          tunnel: w464 -> [_ w475]
          tunnel: [w472 w474] -> w462
          tunnel: [w470 w473] -> w460
          frame False {
          }
          frame True {
            n194 = case shown="True" w476 {
              tunnel: w478 -> [w480 w485]
              tunnel: [w480 w484] -> w477
              tunnel: w475 -> [_ w483]
              tunnel: [_ w482] -> w474
              tunnel: [FALSE FALSE] -> w473
              frame False {
              }
              frame True {
                n195 = stacked-sequence {
                  tunnel: w485 -> [_ w491 _]
                  tunnel: [_ w490 _] -> w484
                  tunnel: w483 -> [_ w489 _]
                  tunnel: [_ w488 _] -> w482
                  frame #0 {
                    n196 = local write "阻断通讯"(TRUE ("阻断通讯")) -> ()
                  }
                  frame #1 {
                    w487 = cluster{"地址":u16, "布尔":bool, "名称":string}[] [{"地址"=50, "布尔"=FALSE, "名称"="启动"}, {"地址"=51, "布尔"=TRUE, "名称"="停止"}]  # A写入线圈信息组
                    n197 = call "写入单个线圈.vi"("error in"=w491, "写入线圈信息组"=w487, "MB_实体"=w489) -> ("输出簇"=w490:errorcluster, "连接成功"=w488:bool)  [unwired: 7 in]
                  }
                  frame #2 {
                    n198 = local write "阻断通讯"(FALSE ("阻断通讯")) -> ()
                  }
                }
              }
            }
          }
        }
        n199 = Bundle By Name(cluster=w463, "正在运行"=w460, "连接成功"=w462) -> (w461:T7)
        n200 = call <vilib>:"Add State(s) to Queue__jki_lib_state_machine.vi"("State(s) in (\"\")"=w469) -> ("States Out"=w468:string)  [unwired: 14 in]
      }
      frame "Communication: 读运行标志" {
        n201 = Unbundle By Name(w494) -> ("serial master instance"=w493:refnum<class "Modbus Master.lvclass">)
        n202 = stacked-sequence {
          tunnel: w499 -> [_ w508 _]
          tunnel: [_ w507 _] -> w498
          tunnel: [_ w506 _] -> w497
          tunnel: [_ w505 _] -> w496
          tunnel: w493 -> [_ w503 _]
          frame #0 {
            n203 = local write "阻断通讯"(TRUE ("阻断通讯")) -> ()
          }
          frame #1 {
            w504 = T9 [{"地址"=507, "数量"=1, "名称"="1测试结束标志", "线圈组"=[]}]  # A读多组线圈信息组
            n204 = call "读线圈组.vi"("error in"=w508, "读多组线圈__输入"=w504, "MB_实体"=w503) -> ("输出簇"=w507:errorcluster, "正在运行"=w505:bool, "连接成功"=w506:bool)  [unwired: 6 in]
          }
          frame #2 {
            n205 = local write "阻断通讯"(FALSE ("阻断通讯")) -> ()
          }
        }
        n206 = Bundle By Name(cluster=w494, "连接成功"=w497, "正在运行"=w496) -> (w495:T7)
        n207 = call <vilib>:"Add State(s) to Queue__jki_lib_state_machine.vi"("State(s) in (\"\")"=w501) -> ("States Out"=w500:string)  [unwired: 14 in]
      }
      frame "---------- 设备状态采集 ----------" {
        # "Do not put any code in this frame.\n(it is a separator no-op)"
        n208 = call <vilib>:"Add State(s) to Queue__jki_lib_state_machine.vi"("State(s) in (\"\")"=w513) -> ("States Out"=w512:string)  [unwired: 14 in]
      }
      frame "通讯参数设置" {
        n209 = stacked-sequence {
          tunnel: w515 -> [_ w523 _]
          tunnel: [_ w520 _] -> w514
          frame #0 {
            n210 = local write "阻断通讯"(TRUE ("阻断通讯")) -> ()
          }
          frame #1 {
            n211 = call "通讯参数设置.vi"() -> ("A设备簇"=w524:T8)  [unwired: 5 in]
            n212 = Unbundle By Name(w524) -> ("MB_实体"=w522:refnum<class "Modbus Master.lvclass">, "连接成功"=w521:bool)
            n213 = Bundle By Name(cluster=w523, "serial master instance"=w522, "连接成功"=w521) -> (w520:T7)
          }
          frame #2 {
            n214 = local write "阻断通讯"(FALSE ("阻断通讯")) -> ()
          }
        }
        n215 = call <vilib>:"Add State(s) to Queue__jki_lib_state_machine.vi"("State(s) in (\"\")"=w518) -> ("States Out"=w517:string)  [unwired: 14 in]
      }
    }
  }
